vi "ContMain.vi"(4 "CtrlRefsin":T4, 5 "Aux chart ref in":refnum<vi>, 6 "steps":i32, 7 "slider refs in":T3, 8 "kinetic img size":cluster{"xpixels":i32, "ypixels":i32}, 9 "File Paths":T5={"Local Save Path"=path "\\\\smbhome.uscs.susx.ac.uk\\cv222/Desktop/data", "Newton Save Path"=path "Z:/#Projects/Entanglement/data", "File Name"="test", "LocalSave"=TRUE}, 10 "Compiler Settings":T6={"Python Path"=path "", "Main File"="makesequence.py", "Meta File"="makesequence.py", "Aux File"="makesequence.py", "Pre File"="metascript.txt"}, 11 "ControllerSettingsRef":refnum<vi>) -> ()   [LabVIEW 2019]
uses:
  PulseCompiler/CompilerSettings.ctl
  controls/FilePaths.ctl
  controls/CompCoilControl.ctl
  controls/FluoSettings.ctl
  controls/xAOMSettings/XAOMsetting.xctl
  controls/PowerStableSettings.ctl
  controls/ControllerSettings.ctl
  PulseControl.ctl
  Compiler/Params.ctl
  Qalibrate/qalibrate.vi
  controls/GlobalExp.vi
  Global.lvlib
panel:
  out "string seq out":string
  out "calib":bool
  out "Pre Sequence":bool
  out "Pre Pulse Seq":T1
  # "Current lock :"
  # "Unlock if :"
  # "Probability lock :"
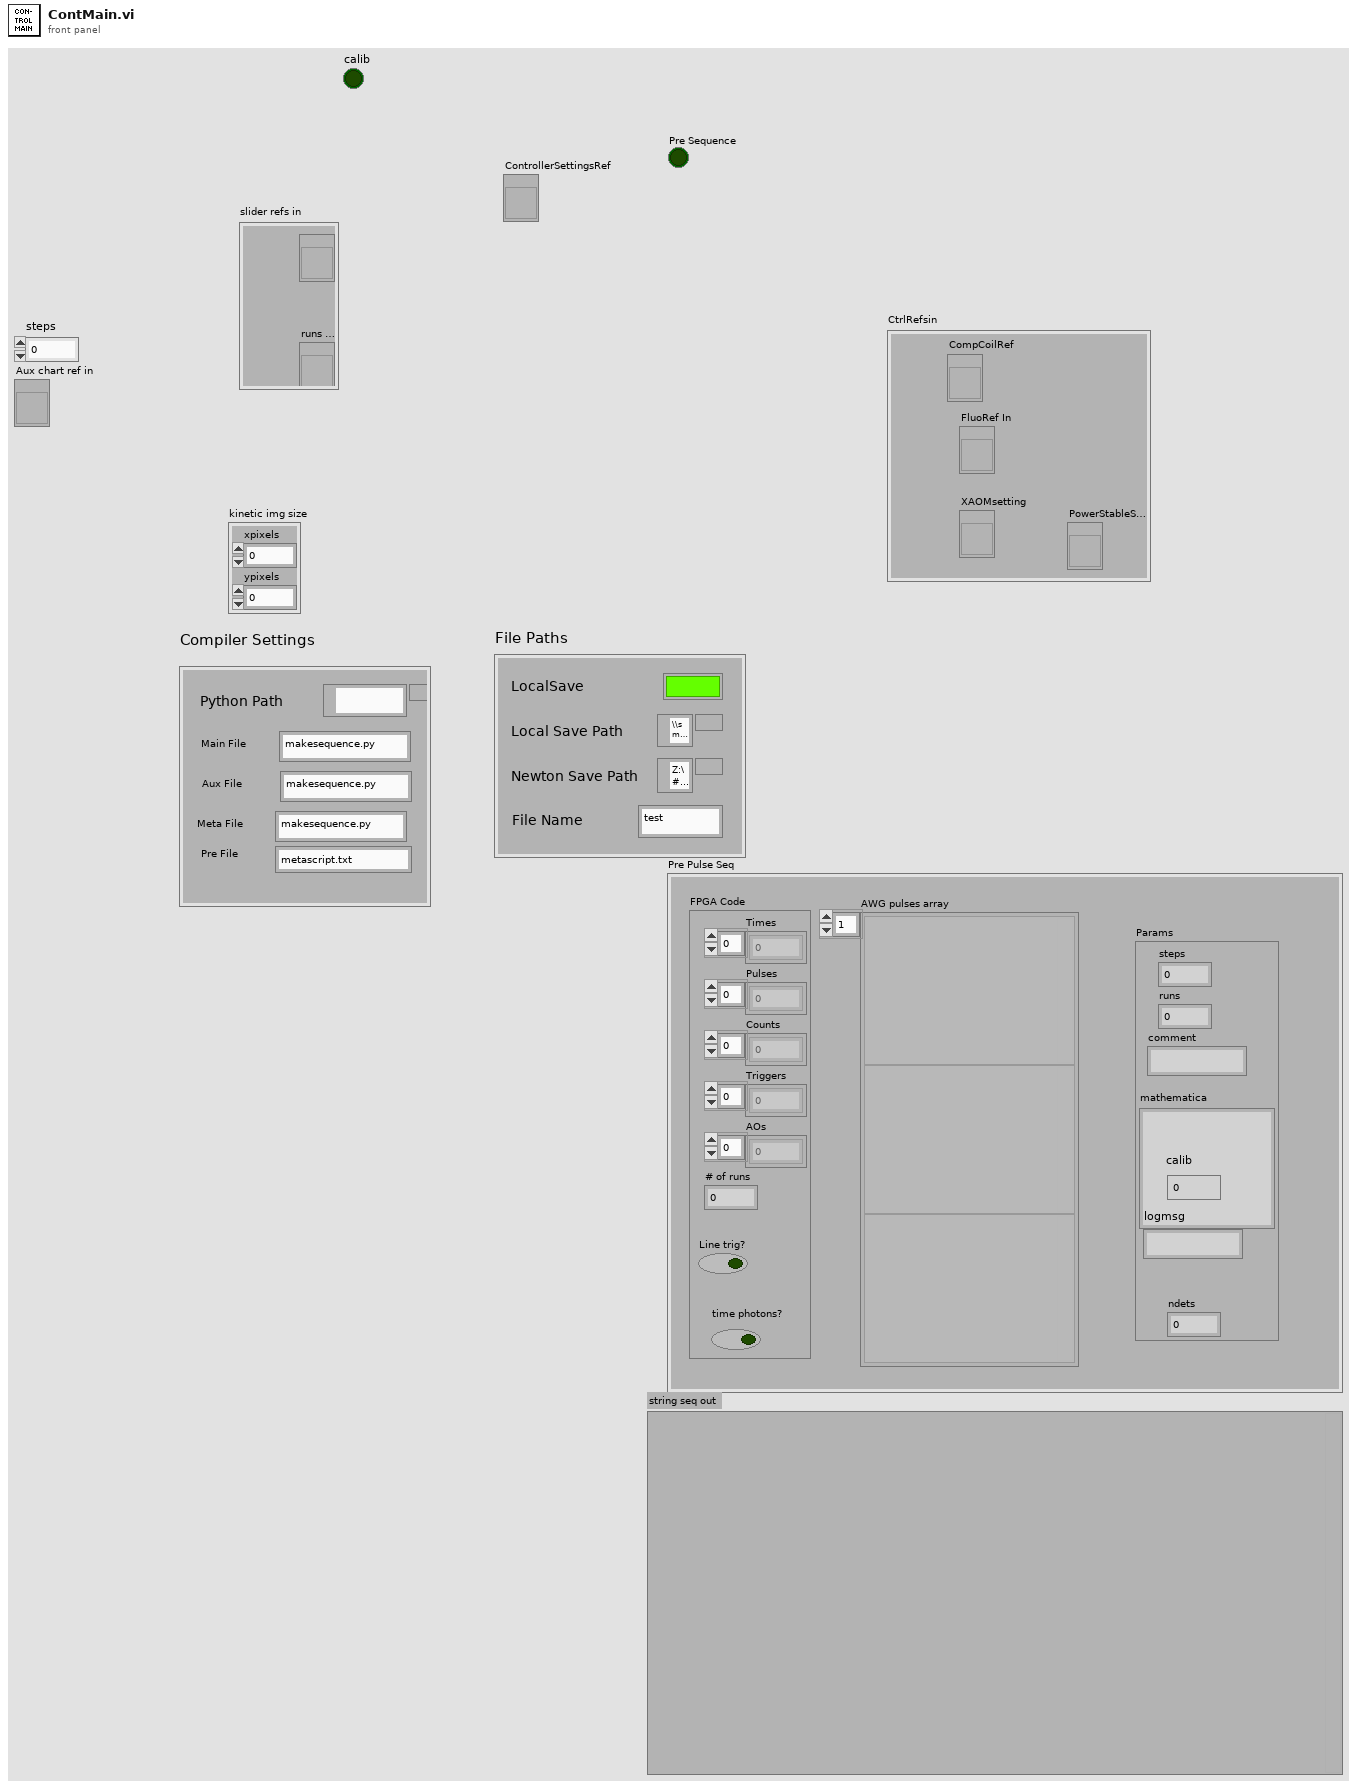
[diagram p1: front panel]
types:
  T1 = typedef "PulseControl.ctl" = cluster{"FPGA Code":cluster{"Times":u32[], "Pulses":u64[], "Counts":u8[], "Triggers":u8[], "AOs":u8[], "# of runs":i32, "Line trig?":bool, "time photons?":bool}, "AWG pulses array":variant[], "Params":T2}
  T2 = typedef "Params.ctl" = cluster{"steps":i16, "runs":i16, "comment":string, "mathematica":string, "calib":i8, "logmsg":string, "ndets":i16}
  T3 = cluster{"steps slider ref":refnum<vi>, "runs slider ref":refnum<vi>}
  T4 = cluster{"CompCoilRef":refnum<vi>, "FluoRef In":refnum<vi>, "XAOMsetting":refnum<vi>, "PowerStableSettings 2":refnum<vi>}
  T5 = typedef "FilePaths.ctl" = cluster{"Local Save Path":path, "Newton Save Path":path, "File Name":string, "LocalSave":bool}
  T6 = typedef "CompilerSettings.ctl" = cluster{"Python Path":path, "Main File":string, "Meta File":string, "Aux File":string, "Pre File":string}
  T7 = enum16{"Innit", "Stop", "Idle", "MainRunning", "AuxRunning"}
  T8 = typedef "ControllerSettings.ctl" = cluster{"Aux Sequence":bool, "Camera":bool, "Recrystallize":bool, "Raw graph":bool, "Mean graph":bool, "Calculate probs":bool, "Find fit":bool, "ReX Time [s] :":dbl, "Lock Voltage :":dbl, "Line trig ":bool, "Check Fluo":bool, "Pre Sequence":bool}
  T9 = cluster{"readout":u32[][], "kinetic series data":i32[][][][], "camera dim":cluster{i32, i32, i32, i32}}
  T10 = cluster{"readout out 2":dbl[][], "kinetic series data":i32[][][][], "camera dim":cluster{i32, i32, i32, i32}}
  T11 = typedef "MasterExpControl.ctl" = cluster{"Main Steps":dbl, "Main Runs":dbl, "ExpStatus":enum16{"Innit", "Stop", "Idle", "MainRunning", "AuxRunning"}, "Main Current Step":dbl, "ExpNum":dbl, "NewData":bool, "date":string, "command":string, "Stop":bool, "Pause":bool, "Mathematica":string, "Main/Meta":bool, "UpdateMath":bool, "Camera":bool, "MetaExpOver":bool, "NextMetaExp":bool}
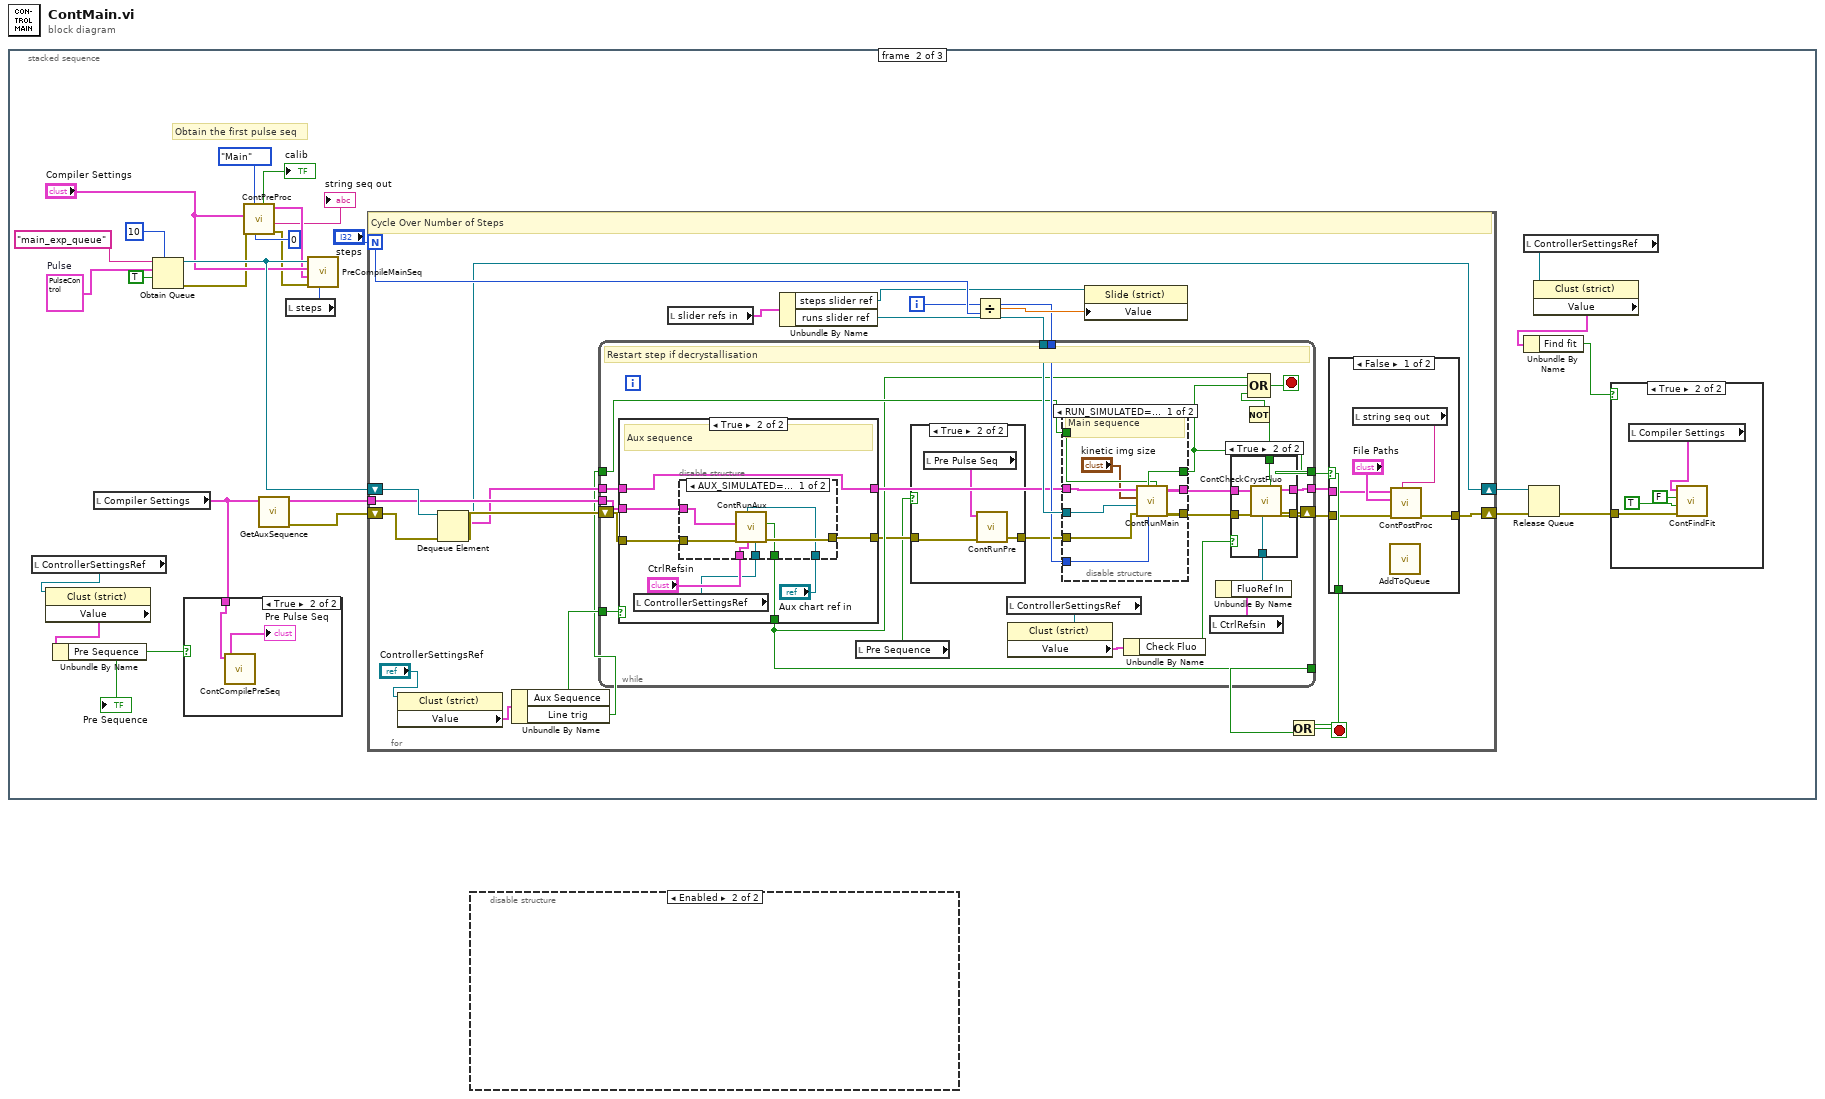
[diagram p0: block diagram]
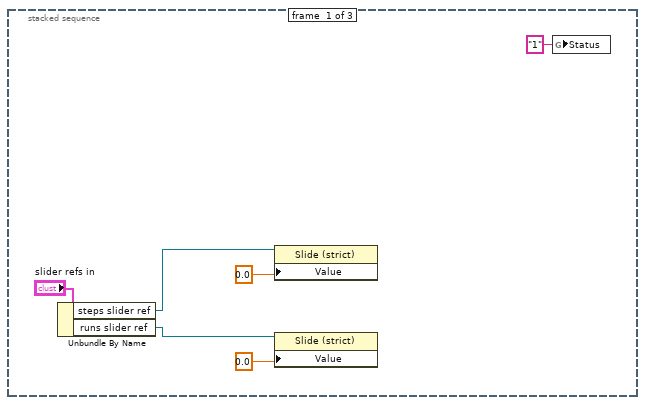
[diagram p2: hidden frame]
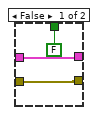
[diagram p6: hidden frame]
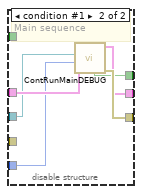
[diagram p7: hidden frame]
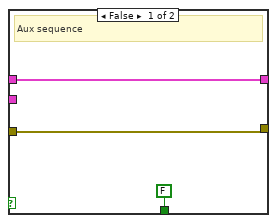
[diagram p8: hidden frame]
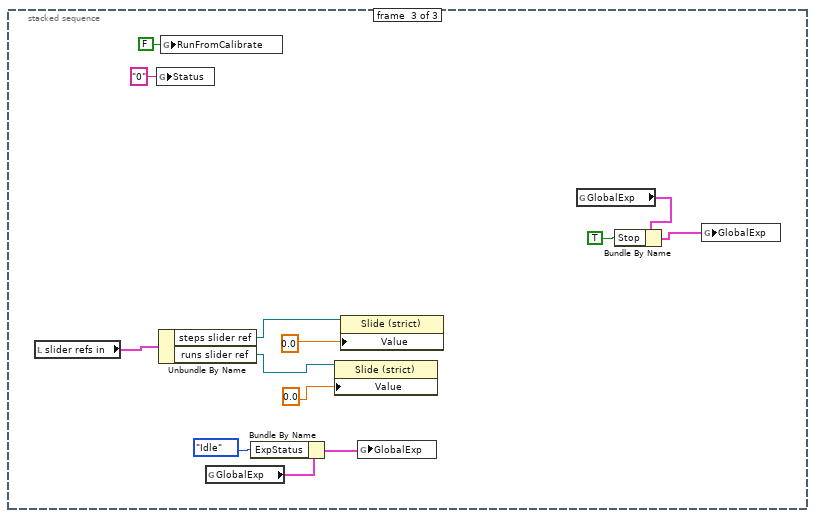
[diagram p11: hidden frame]
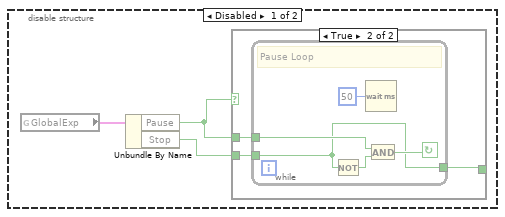
[diagram p12: hidden frame]
diagram:
  n1 = stacked-sequence {
    frame #0 {
      n2 = Unbundle By Name("slider refs in") -> ("steps slider ref"=w3:refnum<vi>, "runs slider ref"=w2:refnum<vi>)
      n3 = property class="Slide (strict)"(reference=w3, "Value"=0.0) -> ()  [unwired: 1 in, 2 out]
      n4 = property class="Slide (strict)"(reference=w2, "Value"=0.0) -> ()  [unwired: 1 in, 2 out]
      n5 = global write "qalibrate.vi" "Status"("1" ("Status")) -> ()
    }
    frame #1 {
      w29 = T1 {"FPGA Code"={"Times"=[], "Pulses"=[], "Counts"=[], "Triggers"=[], "AOs"=[], "# of runs"=0, "Line trig?"=FALSE, "time photons?"=FALSE}, "AWG pulses array"=[], "Params"={"steps"=0, "runs"=0, "comment"="", "mathematica"="", "calib"=0, "logmsg"="", "ndets"=0}}  # Pulse
      # "Obtain the first pulse seq"
      n6 = local read "ControllerSettingsRef"() -> (w18:refnum<vi>)
      n7 = property class="Clust (strict)"(reference=w18) -> ("Value"=w17:T8)  [unwired: 1 in, 2 out]
      n8 = Unbundle By Name(w17) -> ("Pre Sequence"=w16:bool)
      "Pre Sequence" <- w16
      n9 = local read "Compiler Settings"() -> (w19:T6)
      n10 = Obtain Queue(max queue size (-1, unlimited)=10, name (unnamed)="main_exp_queue", element data type=w29, create if not found? (T)=TRUE) -> (queue out=w24:refnum<queue>, error out=w11:errorcluster)  [unwired: 1 in, 1 out]
      n11 = case shown="True" w16 {
        tunnel: w19 -> [_ w35]
        frame False {
        }
        frame True {
          n12 = call "ContCompilePreSeq.vi"("Compiler Settings In"=w35) -> ("Pre Pulse Seq"=→"Pre Pulse Seq":T1)  [unwired: 10 in]
        }
      }
      n13 = call "ContPreProc.vi"("step num"=0, "error in (no error)"=w11, "Compiler Settings"="Compiler Settings", "Enum"=enum16{"Meta", "Aux", "Main"}."Main") -> ("error out"=w10:errorcluster, "string seq out"=→"string seq out":string, "Main pulse seq"=w9:T1, "calib"=→"calib":bool)  [unwired: 3 in, 1 out]
      n14 = call "GetAuxSequence.vi"("Compiler Settings"=w19) -> ("error out"=w27:errorcluster, "Aux Pulse"=w32:T1)  [unwired: 9 in]
      n15 = local read "steps"() -> (w23:i32)
      n16 = call "PreCompileMainSeq.vi"("steps"=w23, "error in (no error)"=w10, "first seq"=w9, "Compiler Settings"="Compiler Settings", "queue in"=w24) -> ()  [unwired: 6 in, 1 out]
      n17 = for {
        N: "steps" -> [w61]
        shift-right: [w48] -> w25
        shift-left: w27 -> [w54]
        tunnel: w32 -> [w52]
        shift-right: [w49] -> w26
        shift-left: w24 -> [w53]
        i -> [w55]
        stop <- w47 stop-if-true
        # "Cycle Over Number of Steps"
        n18 = property class="Clust (strict)"(reference="ControllerSettingsRef") -> ("Value"=w44:T8)  [unwired: 1 in, 2 out]
        n19 = Dequeue Element(queue=w53, error in (no error)=w54) -> (queue out=w49:refnum<queue>, element=w50:T1, error out=w51:errorcluster)  [unwired: 1 in, 1 out]
        n20 = Unbundle By Name(w44) -> ("Aux Sequence"=w57:bool, "Line trig"=w42:bool)
        n21 = local read "slider refs in"() -> (w58:T3)
        n22 = Unbundle By Name(w58) -> ("steps slider ref"=w60:refnum<vi>, "runs slider ref"=w59:refnum<vi>)
        n23 = while {
          tunnel: w59 -> [w87]
          tunnel: w55 -> [w85]
          tunnel: w52 -> [w84]
          tunnel: w50 -> [w82]
          tunnel: [w76] -> w40
          shift-right: [w77] -> w41
          shift-left: w51 -> [w83]
          tunnel: w42 -> [w80]
          tunnel: [w72] -> w56
          tunnel: w57 -> [w86]
          tunnel: [w71] -> w45
          stop <- w74 stop-if-true
          # "Restart step if decrystallisation"
          n24 = case shown="True" w86 {
            tunnel: w84 -> [_ w125]
            tunnel: w83 -> [w118 w124]
            tunnel: w82 -> [w119 w123]
            tunnel: [w119 w123] -> w81
            tunnel: [w118 w122] -> w65
            tunnel: [FALSE ("Aux stopped") w121] -> w71
            frame False {
              # "Aux sequence"
            }
            frame True {
              # "Aux sequence"
              n25 = local read "ControllerSettingsRef"() -> (w120:refnum<vi>)
              n26 = disable-structure shown="AUX_SIMULATED==FALSE" {
                disable-tunnel: [w134 _] -> w122
                disable-tunnel: "Aux chart ref in" -> [w133 _]
                disable-tunnel: "CtrlRefsin" -> [w132 _]
                disable-tunnel: w125 -> [w131 _]
                disable-tunnel: w124 -> [w130 _]
                disable-tunnel: [w129 _] -> w121
                disable-tunnel: w120 -> [w128 _]
                frame condition #0 (active) {
                  n27 = call "ContRunAux.vi"("ControllerSettingsRef"=w128, "CtrlRefsin"=w132, "Aux chart ref in"=w133, "error in (no error)"=w130, "Aux pulse in"=w131) -> ("error out"=w134:errorcluster, "Aux stopped"=w129:bool)  [unwired: 4 in, 1 out]
                }
                frame condition #1 {
                }
              }
            }
          }
          n28 = local read "Pre Sequence"() -> (w63:bool)
          n29 = case shown="True" w63 {
            tunnel: w65 -> [w88 w91]
            tunnel: [w88 w90] -> w64
            frame False {
            }
            frame True {
              n30 = local read "Pre Pulse Seq"() -> (w89:T1)
              n31 = call "ContRunPre.vi"("error in"=w91, "Pre Pulse In"=w89) -> ("error out"=w90:errorcluster)  [unwired: 9 in]
            }
          }
          n32 = local read "ControllerSettingsRef"() -> (w68:refnum<vi>)
          n33 = property class="Clust (strict)"(reference=w68) -> ("Value"=w67:T8)  [unwired: 1 in, 2 out]
          n34 = disable-structure shown="RUN_SIMULATED==FALSE" {
            disable-tunnel: w81 -> [w104 w116]
            disable-tunnel: [w108 w110] -> w79
            disable-tunnel: [w109 w114] -> w78
            disable-tunnel: w87 -> [w106 w113]
            disable-tunnel: [w107 w112] -> w72
            disable-tunnel: w85 -> [w105 w111]
            disable-tunnel: w64 -> [w103 _]
            disable-tunnel: w80 -> [w102 _]
            frame condition #0 (active) {
              # "Main sequence"
              n35 = call "ContRunMain.vi"("line trig"=w102, "Step Number"=w105, "error in"=w103, "runs slider ref"=w106, "image size"="kinetic img size", "Main Pulse In"=w104) -> ("error out"=w109:errorcluster, "readout"=w108:T9, "Stop"=w107:bool)  [unwired: 3 in]
            }
            frame condition #1 {
              # "Main sequence"
              n36 = call "ContRunMainDEBUG.vi"("step num"=w111, "runs slider ref"=w113, "Main pulse seq"=w116) -> ("error out"=w114:errorcluster, "readout"=w110:T10, "Stop"=w112:bool, "error in (no error)"=w115:errorcluster)  [unwired: 5 in]
            }
          }
          n37 = Unbundle By Name(w67) -> ("Check Fluo"=w66:bool)
          n38 = local read "CtrlRefsin"() -> (w70:T4)
          n39 = Unbundle By Name(w70) -> ("FluoRef In"=w69:refnum<vi>)
          n40 = case shown="True" w66 {
            tunnel: w79 -> [w94 w100]
            tunnel: w78 -> [w93 w99]
            tunnel: [w93 w98] -> w77
            tunnel: [w94 w97] -> w76
            tunnel: [FALSE ("restart step?") w96] -> w75
            tunnel: w69 -> [_ w95]
            frame False {
            }
            frame True {
              n41 = call "ContCheckCrystFluo.vi"("FluoRef In"=w95, "error in (no error)"=w99, "readout"=w100) -> ("error out"=w98:errorcluster, "readout 2"=w97:T9, "restart step?"=w96:bool)  [unwired: 6 in]
            }
          }
          n42 = Not(x=w75) -> (.not. x?=w73:bool)
          n43 = Compound Arithmetic op=OR(w71, w72, w73) -> (w74:bool)
        }
        n44 = Divide(x=w55, y=w61) -> (x/y=w62:dbl)
        n45 = property class="Slide (strict)"(reference=w60, "Value"=w62) -> ()  [unwired: 1 in, 2 out]
        n46 = case shown="False" w56 {
          selector: w56 -> [w140 w142]
          tunnel: w41 -> [w137 w141]
          tunnel: [w136 w141] -> w48
          tunnel: [w140 w142] -> w46
          tunnel: w40 -> [w138 _]
          frame False {
            n47 = local read "string seq out"() -> (w135:string)
            n48 = call "AddToQueue.vi"() -> ()  [unwired: 11 in, 1 out]
            n49 = call "ContPostProc.vi"("string seq in"=w135, "Error In"=w137, "File Paths"="File Paths", "readout"=w138) -> ("error out"=w136:errorcluster)  [unwired: 7 in]
          }
          frame True {
          }
        }
        n50 = Or(x=w46, y=w45) -> (x .or. y?=w47:bool)
      }
      n51 = local read "ControllerSettingsRef"() -> (w22:refnum<vi>)
      n52 = Release Queue(queue=w26, error in (no error)=w25) -> (error out=w7:errorcluster)  [unwired: 1 in, 2 out]
      n53 = property class="Clust (strict)"(reference=w22) -> ("Value"=w21:T8)  [unwired: 1 in, 2 out]
      n54 = Unbundle By Name(w21) -> ("Find fit"=w20:bool)
      n55 = case shown="True" w20 {
        tunnel: w7 -> [_ w37]
        frame False {
        }
        frame True {
          n56 = local read "Compiler Settings"() -> (w38:T6)
          n57 = call "ContFindFit.vi"("error in (no error)"=w37, "GenImage"=TRUE, "update"=FALSE, "Compiler Settings"=w38) -> ()  [unwired: 7 in, 1 out]
        }
      }
    }
    frame #2 {
      n58 = local read "slider refs in"() -> (w147:T3)
      n59 = global write "qalibrate.vi" "Status"("0" ("Status")) -> ()
      n60 = Unbundle By Name(w147) -> ("steps slider ref"=w146:refnum<vi>, "runs slider ref"=w145:refnum<vi>)
      n61 = global write "qalibrate.vi" "RunFromCalibrate"(FALSE ("RunFromCalibrate")) -> ()
      n62 = global read "GlobalExp.vi" "GlobalExp"() -> (w152:T11)
      n63 = Bundle By Name(cluster=w152, "ExpStatus"=T7."Idle") -> (w151:T11)
      n64 = property class="Slide (strict)"(reference=w145, "Value"=0.0) -> ()  [unwired: 1 in, 2 out]
      n65 = property class="Slide (strict)"(reference=w146, "Value"=0.0) -> ()  [unwired: 1 in, 2 out]
      n66 = global write "GlobalExp.vi" "GlobalExp"(w151) -> ()
      n67 = global read "GlobalExp.vi" "GlobalExp"() -> (w155:T11)
      n68 = Bundle By Name(cluster=w155, "Stop"=TRUE) -> (w154:T11)
      n69 = global write "GlobalExp.vi" "GlobalExp"(w154) -> ()
    }
  }
  n70 = disable-structure shown="Enabled" {
    frame Disabled {
      n71 = global read "GlobalExp.vi" "GlobalExp"() -> (w158:T11)
      n72 = Unbundle By Name(w158) -> ("Pause"=w157:bool, "Stop"=w156:bool)
      n73 = case shown="True" w157 {
        tunnel: w157 -> [_ w162]
        tunnel: w156 -> [w159 w161]
        tunnel: [w159 w160] -> _
        frame False {
        }
        frame True {
          n74 = while {
            tunnel: w162 -> [w164]
            tunnel: w161 -> [w163]
            tunnel: [w163] -> w160
            stop <- w166 continue-if-true
            # "Pause Loop"
            n75 = Not(x=w163) -> (.not. x?=w165:bool)
            n76 = Wait (ms)(milliseconds to wait=u32 50) -> ()  [unwired: 1 out]
            n77 = And(x=w164, y=w165) -> (x .and. y?=w166:bool)
          }
        }
      }
    }
    frame Enabled {
    }
  }
